vi "LabAssignment4.vi"() -> ()   [LabVIEW 2015]
panel:
  in  "STOP":bool
  in  "START":bool
  in  "Loser":bool
  out "Array 2":dbl[](array[numeric])
  out "Array":dbl[](array[numeric])
  in  "Blue":bool
  in  "Red":bool
  in  "Yellow":bool
  in  "Green":bool
  out "x*y":dbl
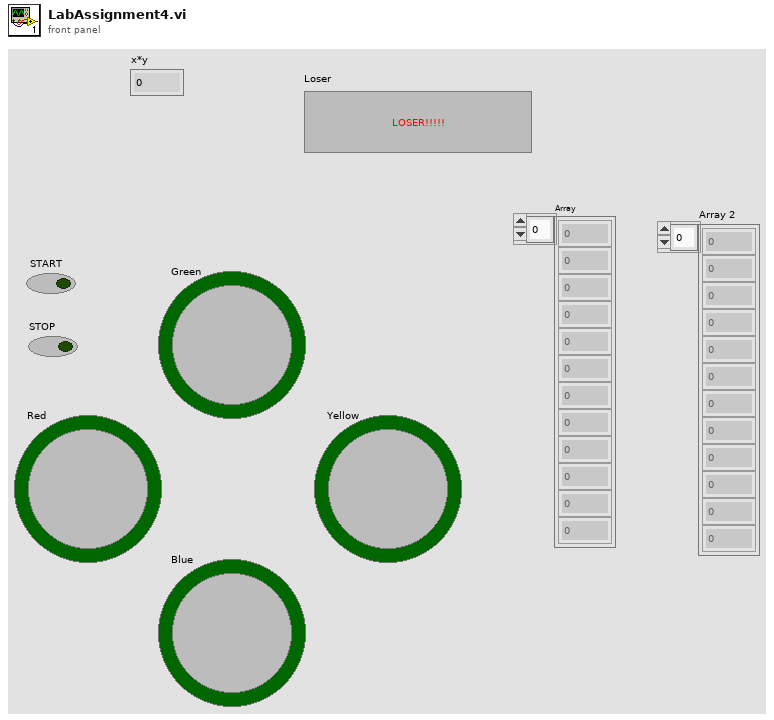
[diagram p1: front panel]
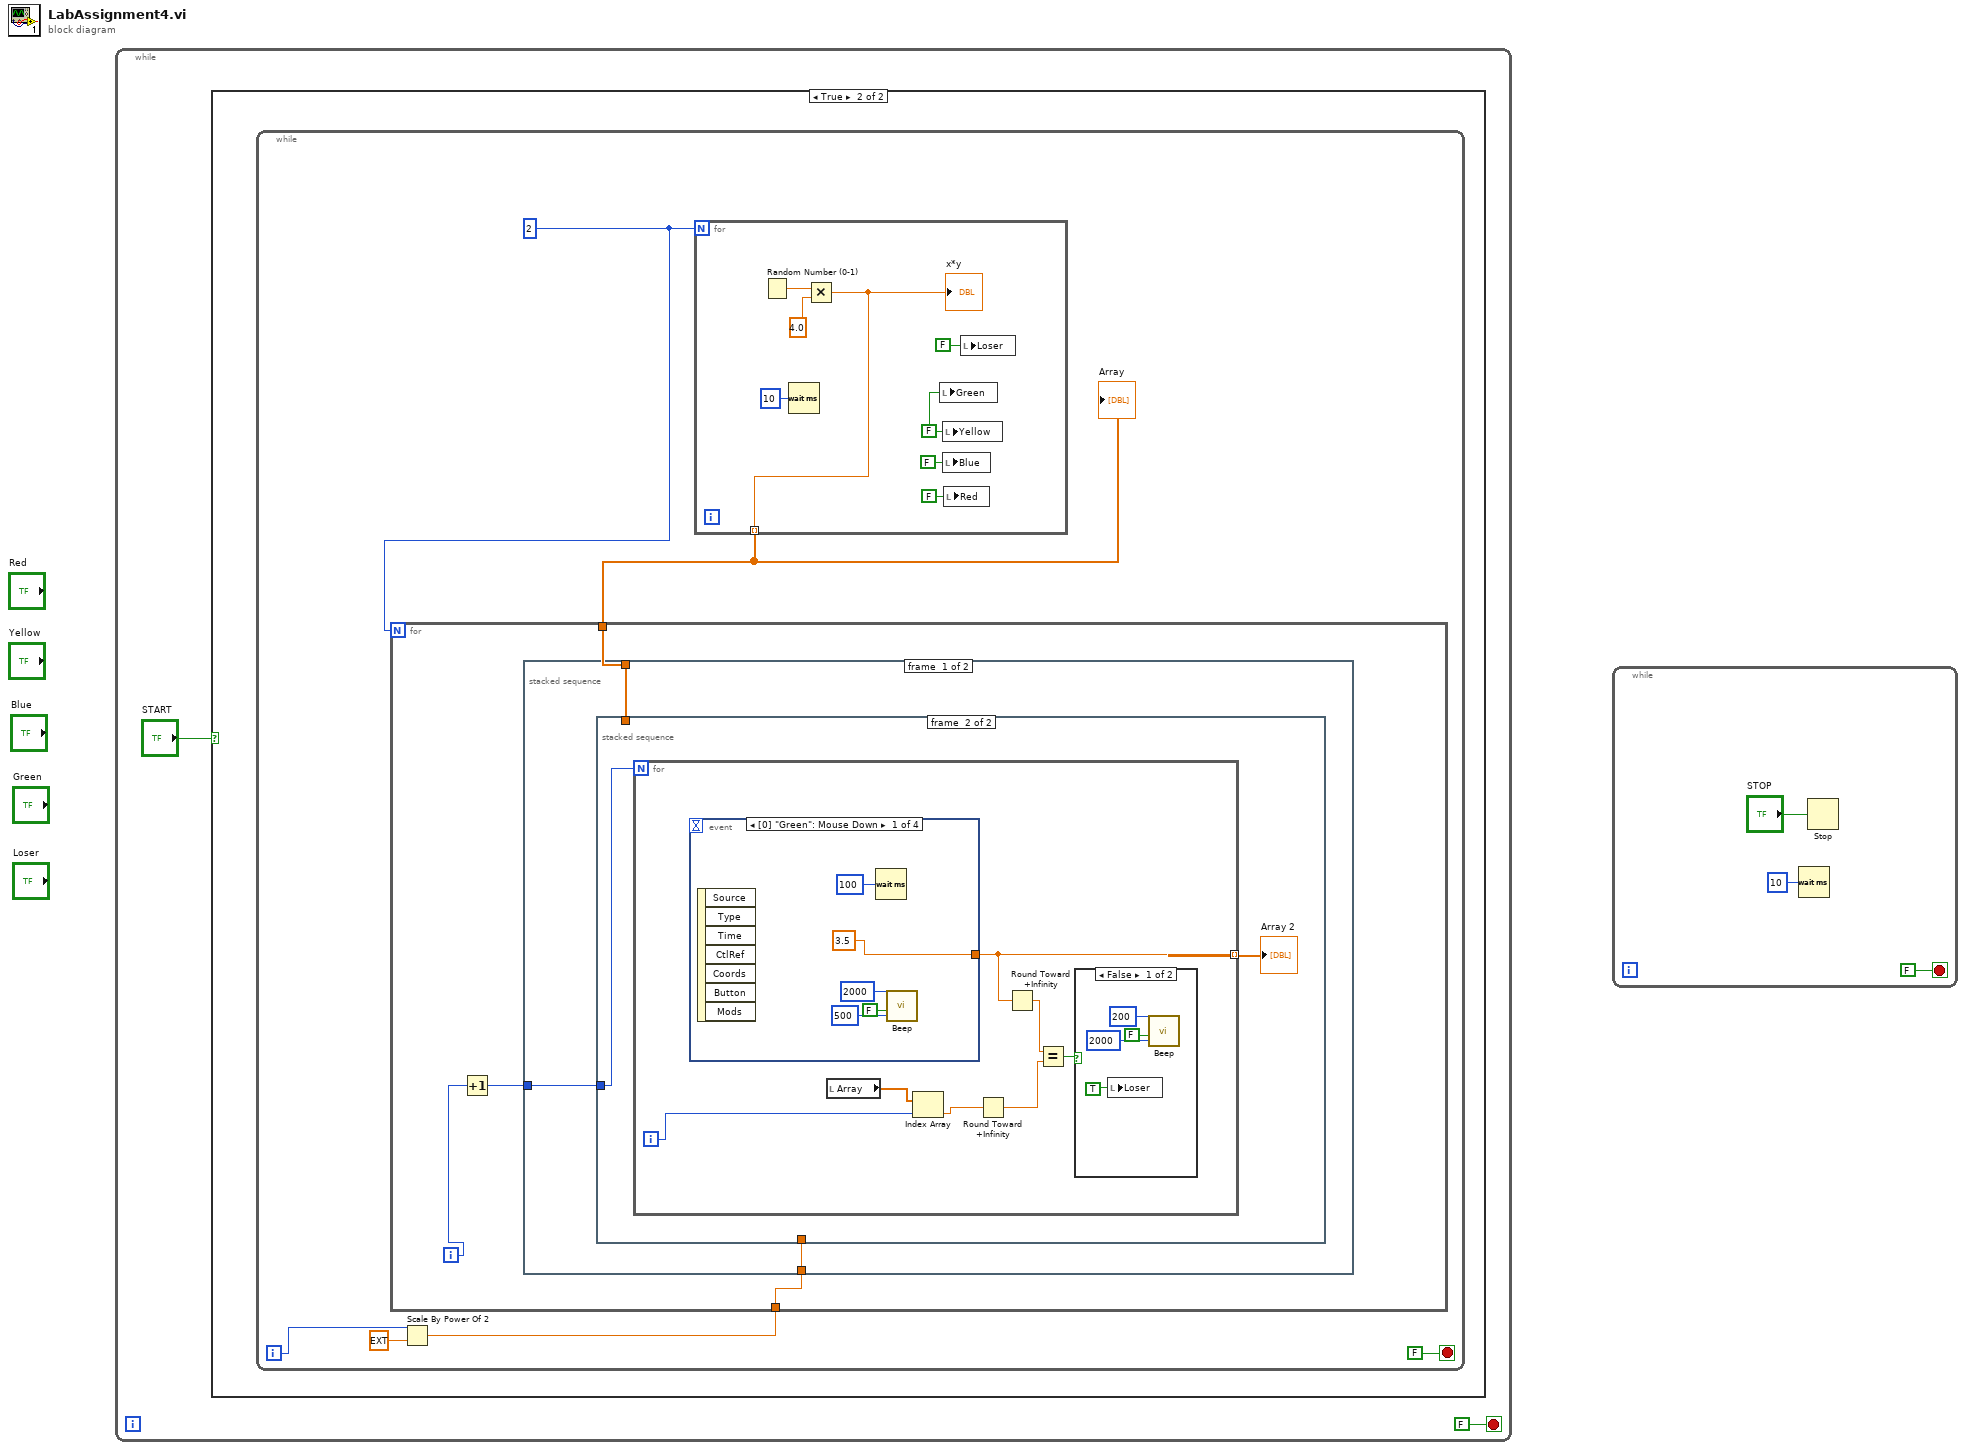
[diagram p0: block diagram]
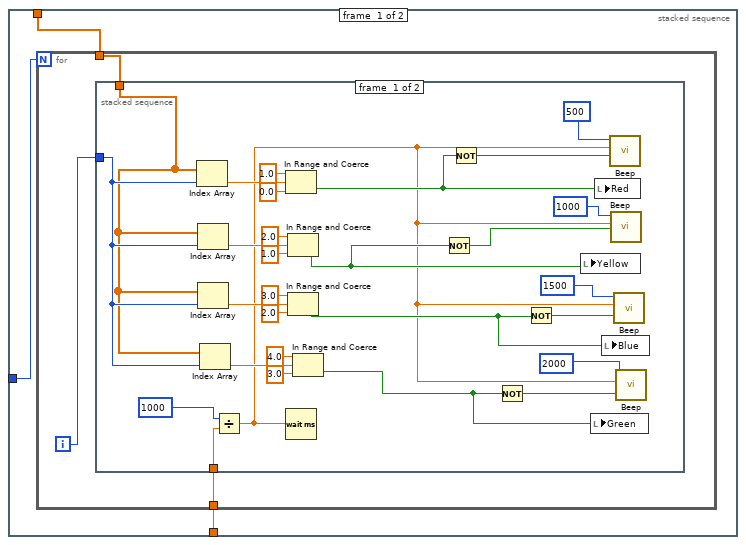
[diagram p3: hidden frame]
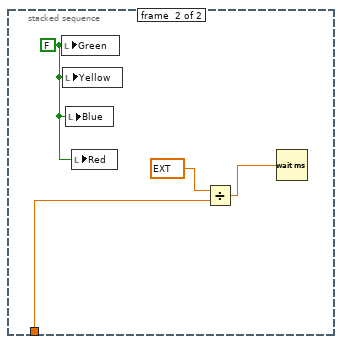
[diagram p4: hidden frame]
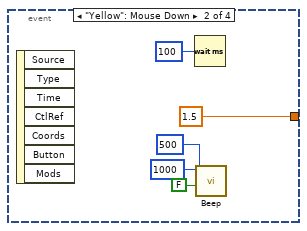
[diagram p6: hidden frame]
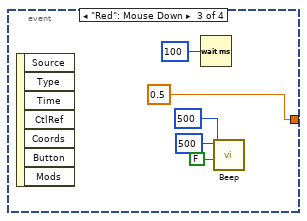
[diagram p7: hidden frame]
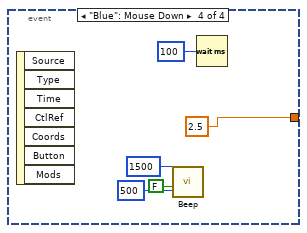
[diagram p8: hidden frame]
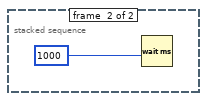
[diagram p9: hidden frame]
diagram:
  n1 = while {
    stop <- FALSE stop-if-true
    n2 = case shown="True" "START" {
      frame False {
      }
      frame True {
        n3 = while {
          i -> [w5]
          stop <- FALSE stop-if-true
          w7 = 2
          n4 = Scale By Power Of 2(n=w5, x=ext 1.0) -> (x*2^n=w3:ext)
          n5 = for {
            N: w7 -> [_]
            tunnel: [w90] -> w8 mode=indexing
            w91 = FALSE ("Yellow")
            n6 = Random Number (0-1)() -> (number: 0 to 1=w95:dbl)
            n7 = Wait (ms)(milliseconds to wait=u32 10) -> ()  [unwired: 1 out]
            n8 = Multiply(x=w95, y=4.0) -> (x*y=w90:dbl)
            "x*y" <- w90
            n9 = local write "Green"(w91) -> ()
            n10 = local write "Yellow"(w91) -> ()
            n11 = local write "Blue"(FALSE ("Blue")) -> ()
            n12 = local write "Red"(FALSE ("Red")) -> ()
            n13 = local write "Loser"(FALSE ("Loser")) -> ()
          }
          "Array" <- w8
          n14 = for {
            N: w7 -> [_]
            tunnel: w8 -> [w10]
            tunnel: w3 -> [w9]
            i -> [w12]
            n15 = Increment(x=w12) -> (x+1=w11:i32)
            n16 = stacked-sequence {
              tunnel: w11 -> [w15 _]
              tunnel: w10 -> [w14 _]
              tunnel: w9 -> [w13 _]
              frame #0 {
                n17 = stacked-sequence {
                  tunnel: w14 -> [w18 _]
                  tunnel: w15 -> [w17 w56]
                  tunnel: w13 -> [w16 _]
                  frame #0 {
                    n18 = for {
                      N: w17 -> [_]
                      tunnel: w18 -> [w20]
                      tunnel: w16 -> [w19]
                      i -> [w21]
                      n19 = stacked-sequence {
                        tunnel: w21 -> [w38 _]
                        tunnel: w20 -> [w37 _]
                        tunnel: w19 -> [w24 w53]
                        frame #0 {
                          n20 = Index Array(array=w37, index=w38) -> (element=w42:dbl)
                          n21 = Index Array(array=w37, index=w38) -> (element=w41:dbl)
                          n22 = Index Array(array=w37, index=w38) -> (element=w40:dbl)
                          n23 = Index Array(array=w37, index=w38) -> (element=w39:dbl)
                          n24 = Divide(x=u32 1000 ("milliseconds to wait"), y=w24) -> (x/y=w22:ext)
                          n25 = In Range and Coerce(upper limit=1.0, x=w42, lower limit=0.0) -> (In Range?=w31:bool)  [unwired: 1 out]
                          n26 = Wait (ms)(milliseconds to wait=w22) -> ()  [unwired: 1 out]
                          n27 = In Range and Coerce(upper limit=2.0, x=w41, lower limit=1.0) -> (In Range?=w30:bool)  [unwired: 1 out]
                          n28 = In Range and Coerce(upper limit=3.0, x=w40, lower limit=2.0) -> (In Range?=w27:bool)  [unwired: 1 out]
                          n29 = In Range and Coerce(upper limit=4.0, x=w39, lower limit=3.0) -> (In Range?=w26:bool)  [unwired: 1 out]
                          n30 = Not(x=w30) -> (.not. x?=w29:bool)
                          n31 = Not(x=w31) -> (.not. x?=w32:bool)
                          n32 = Not(x=w26) -> (.not. x?=w25:bool)
                          n33 = Not(x=w27) -> (.not. x?=w28:bool)
                          n34 = local write "Yellow"(w30) -> ()
                          n35 = local write "Green"(w26) -> ()
                          n36 = local write "Red"(w31) -> ()
                          n37 = local write "Blue"(w27) -> ()
                          n38 = call <vilib>:"Beep.vi"("use system alert? (T)"=w32, "duration (msec)"=w22, "frequency (Hz)"=u32 500) -> ()  [unwired: 9 in]
                          n39 = call <vilib>:"Beep.vi"("use system alert? (T)"=w29, "duration (msec)"=w22, "frequency (Hz)"=u32 1000) -> ()  [unwired: 9 in]
                          n40 = call <vilib>:"Beep.vi"("use system alert? (T)"=w28, "duration (msec)"=w22, "frequency (Hz)"=u32 1500) -> ()  [unwired: 9 in]
                          n41 = call <vilib>:"Beep.vi"("use system alert? (T)"=w25, "duration (msec)"=w22, "frequency (Hz)"=u32 2000) -> ()  [unwired: 9 in]
                        }
                        frame #1 {
                          w54 = FALSE ("Green")
                          n42 = local write "Green"(w54) -> ()
                          n43 = local write "Yellow"(w54) -> ()
                          n44 = local write "Blue"(w54) -> ()
                          n45 = local write "Red"(w54) -> ()
                          n46 = Divide(x=ext 1000.0, y=w53) -> (x/y=w51:ext)
                          n47 = Wait (ms)(milliseconds to wait=w51) -> ()  [unwired: 1 out]
                        }
                      }
                    }
                  }
                  frame #1 {
                    n48 = for {
                      N: w56 -> [_]
                      tunnel: [w58] -> w55 mode=indexing
                      i -> [w61]
                      n49 = event shown="[0] \"Green\": Mouse Down" {
                        selector: _ -> [_ _ _ _]
                        dyn-events: _ -> [_ _ _ _]
                        timeout: _ -> [_ _ _ _]
                        tunnel: [3.5 ("element") 1.5 ("element") 0.5 ("element") 2.5 ("element")] -> w58
                        event "Green": Mouse Down {
                          n50 = event-data() -> ()  [unwired: 1 in, 7 out]
                          n51 = Wait (ms)(milliseconds to wait=u32 100) -> ()  [unwired: 1 out]
                          n52 = call <vilib>:"Beep.vi"("use system alert? (T)"=FALSE, "duration (msec)"=u32 500, "frequency (Hz)"=u32 2000) -> ()  [unwired: 9 in]
                        }
                        event "Yellow": Mouse Down {
                          n53 = event-data() -> ()  [unwired: 1 in, 7 out]
                          n54 = Wait (ms)(milliseconds to wait=u32 100) -> ()  [unwired: 1 out]
                          n55 = call <vilib>:"Beep.vi"("use system alert? (T)"=FALSE, "duration (msec)"=u32 500, "frequency (Hz)"=u32 1000) -> ()  [unwired: 9 in]
                        }
                        event "Red": Mouse Down {
                          n56 = event-data() -> ()  [unwired: 1 in, 7 out]
                          n57 = Wait (ms)(milliseconds to wait=u32 100) -> ()  [unwired: 1 out]
                          n58 = call <vilib>:"Beep.vi"("use system alert? (T)"=FALSE, "duration (msec)"=u32 500, "frequency (Hz)"=u32 500) -> ()  [unwired: 9 in]
                        }
                        event "Blue": Mouse Down {
                          n59 = event-data() -> ()  [unwired: 1 in, 7 out]
                          n60 = call <vilib>:"Beep.vi"("use system alert? (T)"=FALSE, "duration (msec)"=u32 500, "frequency (Hz)"=u32 1500) -> ()  [unwired: 9 in]
                          n61 = Wait (ms)(milliseconds to wait=u32 100) -> ()  [unwired: 1 out]
                        }
                      }
                      n62 = local read "Array"() -> (w62:dbl[])
                      n63 = Index Array(array=w62, index=w61) -> (element=w60:dbl)
                      n64 = Round Toward +Infinity(x=w60) -> (ceil(x): smallest int >= x=w63:dbl)
                      n65 = Round Toward +Infinity(x=w58) -> (ceil(x): smallest int >= x=w57:dbl)
                      n66 = Equal?(x=w57, y=w63) -> (x = y?=w59:bool)
                      n67 = case shown="False" w59 {
                        frame False {
                          n68 = local write "Loser"(TRUE ("Loser")) -> ()
                          n69 = call <vilib>:"Beep.vi"("use system alert? (T)"=FALSE, "duration (msec)"=u32 2000, "frequency (Hz)"=u32 200) -> ()  [unwired: 9 in]
                        }
                        frame True {
                        }
                      }
                    }
                    "Array 2" <- w55
                  }
                }
              }
              frame #1 {
                n70 = Wait (ms)(milliseconds to wait=u32 1000) -> ()  [unwired: 1 out]
              }
            }
          }
        }
      }
    }
  }
  n71 = while {
    stop <- FALSE stop-if-true
    n72 = Wait (ms)(milliseconds to wait=u32 10) -> ()  [unwired: 1 out]
    n73 = Stop(stop? (T)="STOP") -> ()
  }
